vi "Get Team Ranking Web.vi"(11 "LabVIEW Web Service Request":refnum<class "Web Request.lvclass">) -> (3 "XML":string)   [LabVIEW 2013]
uses:
  <vilib>/wsapi/Web Request.lvclass
  <vilib>/xml/Close Reference(Node).vi
  <vilib>/xml/NI_XML.lvlib
  <resource>/objmgr/DOMUserDefRef.rc
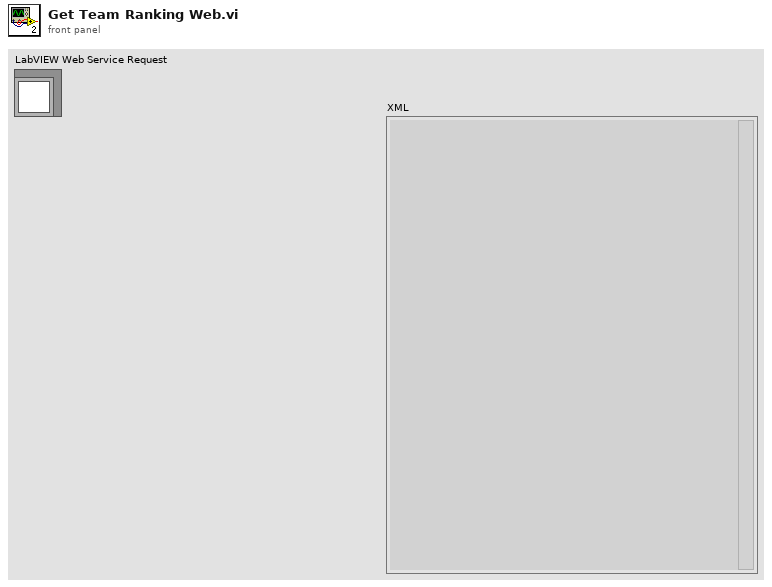
[diagram p1: front panel]
types:
  T1 = enum16{"Get", "Increment", "Decrement", "Set Match", "Set Phase"}
  T2 = cluster{"GUID":u16, "Team Number":u16, "Team Name":string, "Highest Score":dbl, "Scores":cluster{"Score":dbl, "Round":u16}[]}[]
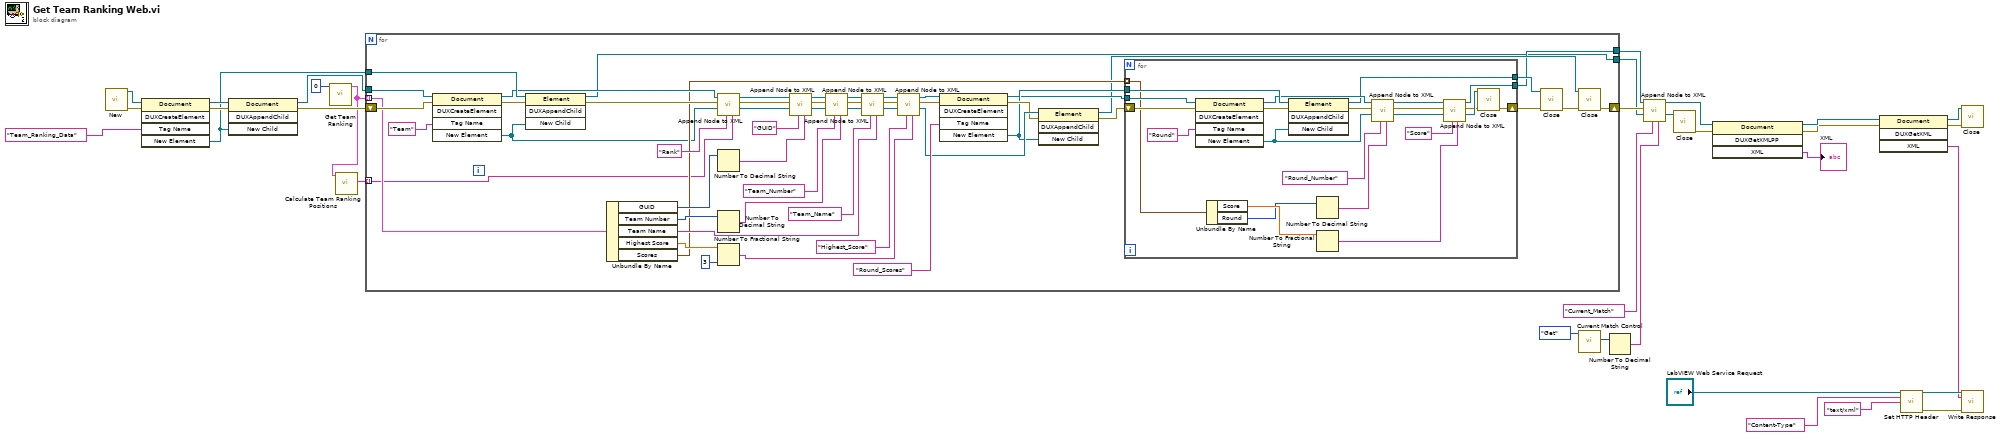
[diagram p0: block diagram]
diagram:
  n1 = call <vilib>:"New.vi"() -> ("error out"=w30:errorcluster, "DOM document out"=w31:refnum<k20>)  [unwired: 8 in]
  n2 = invoke class="Document" method="DUXCreateElement"(reference=w31, error in=w30, "Tag Name"="Team_Ranking_Data") -> (reference out=w28:refnum<k20>, error out=w27:errorcluster, "New Element"=w24:refnum<k20>)  [unwired: 2 in, 2 out]
  n3 = invoke class="Document" method="DUXAppendChild"(reference=w28, error in=w27, "New Child"=w24) -> (reference out=w26:refnum<k20>, error out=w25:errorcluster)  [unwired: 1 in, 2 out]
  n4 = call "Get Team Ranking.vi"("Needed Validations"=u16 0) -> ("Ranked Teams"=w2:T2)  [unwired: 10 in]
  n5 = call "Calculate Team Ranking Positions.vi"("Ranked Teams in"=w2) -> ("Rankings"=w1:string[])  [unwired: 9 in, 1 out]
  n6 = for {
    tunnel: w2 -> [w78] mode=indexing
    tunnel: w26 -> [w83]
    shift-right: [w37] -> w9
    shift-left: w25 -> [w82]
    tunnel: w24 -> [w80]
    tunnel: [w36] -> w11
    tunnel: [w35] -> w8
    tunnel: w1 -> [w33] mode=indexing
    n7 = invoke class="Document" method="DUXCreateElement"(reference=w83, error in=w82, "Tag Name"="Team") -> (reference out=w77:refnum<k20>, error out=w79:errorcluster, "New Element"=w38:refnum<k20>)  [unwired: 2 in, 2 out]
    n8 = invoke class="Element" method="DUXAppendChild"(reference=w80, error in=w79, "New Child"=w38) -> (reference out=w35:refnum<k20>, error out=w76:errorcluster)  [unwired: 1 in, 2 out]
    n9 = Unbundle By Name(w78) -> ("GUID"=w70:u16, "Team Number"=w64:u16, "Team Name"=w58:string, "Highest Score"=w53:dbl, "Scores"=w51:cluster{"Score":dbl, "Round":u16}[])
    n10 = call "Append Node to XML.vi"("Data"=w33, "Tag Name"="Rank", "SuperElement In"=w38, "error in"=w76, "DOM document in"=w77) -> ("SuperElement Out"=w72:refnum<k20>, "error out"=w73:errorcluster, "DOM document out"=w74:refnum<k20>)  [unwired: 4 in]
    n11 = Number To Decimal String(number=w70) -> (decimal integer string=w69:string)  [unwired: 1 in]
    n12 = Number To Decimal String(number=w64) -> (decimal integer string=w63:string)  [unwired: 1 in]
    n13 = Number To Fractional String(number=w53, precision (6)=i16 3) -> (F-format string=w52:string)  [unwired: 2 in]
    n14 = call "Append Node to XML.vi"("Data"=w69, "Tag Name"="GUID", "SuperElement In"=w72, "error in"=w73, "DOM document in"=w74) -> ("SuperElement Out"=w66:refnum<k20>, "error out"=w67:errorcluster, "DOM document out"=w68:refnum<k20>)  [unwired: 4 in]
    n15 = call "Append Node to XML.vi"("Data"=w63, "Tag Name"="Team_Number", "SuperElement In"=w66, "error in"=w67, "DOM document in"=w68) -> ("SuperElement Out"=w60:refnum<k20>, "error out"=w61:errorcluster, "DOM document out"=w62:refnum<k20>)  [unwired: 4 in]
    n16 = call "Append Node to XML.vi"("Data"=w58, "Tag Name"="Team_Name", "SuperElement In"=w60, "error in"=w61, "DOM document in"=w62) -> ("SuperElement Out"=w55:refnum<k20>, "error out"=w56:errorcluster, "DOM document out"=w57:refnum<k20>)  [unwired: 4 in]
    n17 = call "Append Node to XML.vi"("Data"=w52, "Tag Name"="Highest_Score", "SuperElement In"=w55, "error in"=w56, "DOM document in"=w57) -> ("SuperElement Out"=w48:refnum<k20>, "error out"=w47:errorcluster, "DOM document out"=w50:refnum<k20>)  [unwired: 4 in]
    n18 = invoke class="Document" method="DUXCreateElement"(reference=w50, error in=w47, "Tag Name"="Round_Scores") -> (reference out=w43:refnum<k20>, error out=w46:errorcluster, "New Element"=w44:refnum<k20>)  [unwired: 2 in, 2 out]
    n19 = invoke class="Element" method="DUXAppendChild"(reference=w48, error in=w46, "New Child"=w44) -> (reference out=w39:refnum<k20>, error out=w45:errorcluster)  [unwired: 1 in, 2 out]
    n20 = for {
      tunnel: w51 -> [w93] mode=indexing
      shift-right: [w85] -> w41
      shift-left: w45 -> [w102]
      tunnel: w44 -> [w100]
      tunnel: w43 -> [w103]
      tunnel: [w104] -> w36
      tunnel: [w84] -> w42
      n21 = invoke class="Document" method="DUXCreateElement"(reference=w103, error in=w102, "Tag Name"="Round") -> (reference out=w98:refnum<k20>, error out=w99:errorcluster, "New Element"=w97:refnum<k20>)  [unwired: 2 in, 2 out]
      n22 = Unbundle By Name(w93) -> ("Score"=w92:dbl, "Round"=w91:u16)
      n23 = invoke class="Element" method="DUXAppendChild"(reference=w100, error in=w99, "New Child"=w97) -> (reference out=w84:refnum<k20>, error out=w95:errorcluster)  [unwired: 1 in, 2 out]
      n24 = Number To Decimal String(number=w91) -> (decimal integer string=w90:string)  [unwired: 1 in]
      n25 = Number To Fractional String(number=w92) -> (F-format string=w105:string)  [unwired: 3 in]
      n26 = call "Append Node to XML.vi"("Data"=w90, "Tag Name"="Round_Number", "SuperElement In"=w97, "error in"=w95, "DOM document in"=w98) -> ("SuperElement Out"=w88:refnum<k20>, "error out"=w89:errorcluster, "DOM document out"=w94:refnum<k20>)  [unwired: 4 in]
      n27 = call "Append Node to XML.vi"("Data"=w105, "Tag Name"="Score", "SuperElement In"=w88, "error in"=w89, "DOM document in"=w94) -> ("SuperElement Out"=w87:refnum<k20>, "error out"=w86:errorcluster, "DOM document out"=w104:refnum<k20>)  [unwired: 4 in]
      n28 = call-poly <vilib>:"Close.vi"("error in (no error)"=w86, "node"=w87) -> ("error out"=w85:errorcluster)  [unwired: 7 in]
    }
    n29 = call-poly <vilib>:"Close.vi"("error in (no error)"=w41, "node"=w42) -> ("error out"=w40:errorcluster)  [unwired: 7 in]
    n30 = call-poly <vilib>:"Close.vi"("error in (no error)"=w40, "node"=w39) -> ("error out"=w37:errorcluster)  [unwired: 7 in]
  }
  n31 = call "Current Match Control.vi"("Mode"=T1."Get") -> ("Current Match"=w5:u16)  [unwired: 9 in, 1 out]
  n32 = Number To Decimal String(number=w5) -> (decimal integer string=w4:string)  [unwired: 1 in]
  n33 = call "Append Node to XML.vi"("Data"=w4, "Tag Name"="Current_Match", "SuperElement In"=w8, "error in"=w9, "DOM document in"=w11) -> ("SuperElement Out"=w7:refnum<k20>, "DOM document out"=w10:refnum<k20>)  [unwired: 4 in, 1 out]
  n34 = call-poly <vilib>:"Close.vi"("node"=w7) -> ("error out"=w23:errorcluster)  [unwired: 8 in]
  n35 = invoke class="Document" method="DUXGetXMLPP"(reference=w10, error in=w23) -> (reference out=w21:refnum<k20>, error out=w20:errorcluster, "XML"=→"XML":string)  [unwired: 2 in, 1 out]
  n36 = invoke class="Document" method="DUXGetXML"(reference=w21, error in=w20) -> (reference out=w19:refnum<k20>, error out=w18:errorcluster, "XML"=w14:string)  [unwired: 2 in, 1 out]
  n37 = call <vilib>:"Set HTTP Header.vi"("LabVIEW Web Service Request"="LabVIEW Web Service Request", "header"="Content-Type", "header value"="text/xml") -> ("LabVIEW Web Service Request out"=w16:refnum<class "Web Request.lvclass">, "error out"=w15:errorcluster)  [unwired: 11 in]
  n38 = call-poly <vilib>:"Close.vi"("error in (no error)"=w18, "node"=w19) -> ()  [unwired: 7 in, 1 out]
  n39 = call <vilib>:"Write Response.vi"("LabVIEW Web Service Request"=w16, "response string"=w14, "error in (no error)"=w15) -> ()  [unwired: 11 in, 2 out]
